vi "SelectMenu5.vi"(0 "XRef":T19, 1 "Tag":T14, 2 "Point":T17, 3 "Menu Type":T16, 4 "State In":T1) -> (14 "Reply":T13, 15 "Handled?":T15, 16 "Multi Object Popup Options":T12, 17 "Fatal Error Out":T11, 18 "State Out":T1)   [LabVIEW 2020, in "Parallel Diagram Block.xnode"]
uses:
  Parallel Diagram Block.xnode
  <vilib>/XNodeSupport/XNodeXNodeRef.ctl
  <vilib>/XNodeSupport/XNodeString.ctl
  <vilib>/XNodeSupport/XNodePoint.ctl
  <vilib>/XNodeSupport/XNodeInt.ctl
  <vilib>/XNodeSupport/XNodeMenuType.ctl
  State.ctl
  Parallel Block/Type Descriptor.ctl
  Parallel Block/Direction.ctl
  Parallel Block/Value Type.ctl
  Parallel Block/Terminal Mode.ctl
  Parallel Block/Terminal Type.ctl
  Parallel Block/Type Mode.ctl
  Parallel Block/Value Mode.ctl
  <vilib>/picture/picture.llb/imagedata.ctl
  Parallel Block/Manager Node.ctl
  <vilib>/XNodeSupport/XNodeStringArray.ctl
  <vilib>/XNodeSupport/XNodeBool.ctl
  <vilib>/XNodeSupport/XNodeMultiObjectPopupOptions.ctl
  <vilib>/XNodeSupport/XNodeErrorCluster.ctl
  Parallel Block/OpMenu Action.ctl
  Parallel Block/Parallel Block.lvlib
  <vilib>/XNodeSupport/NI_XNodeSupport.lvlib
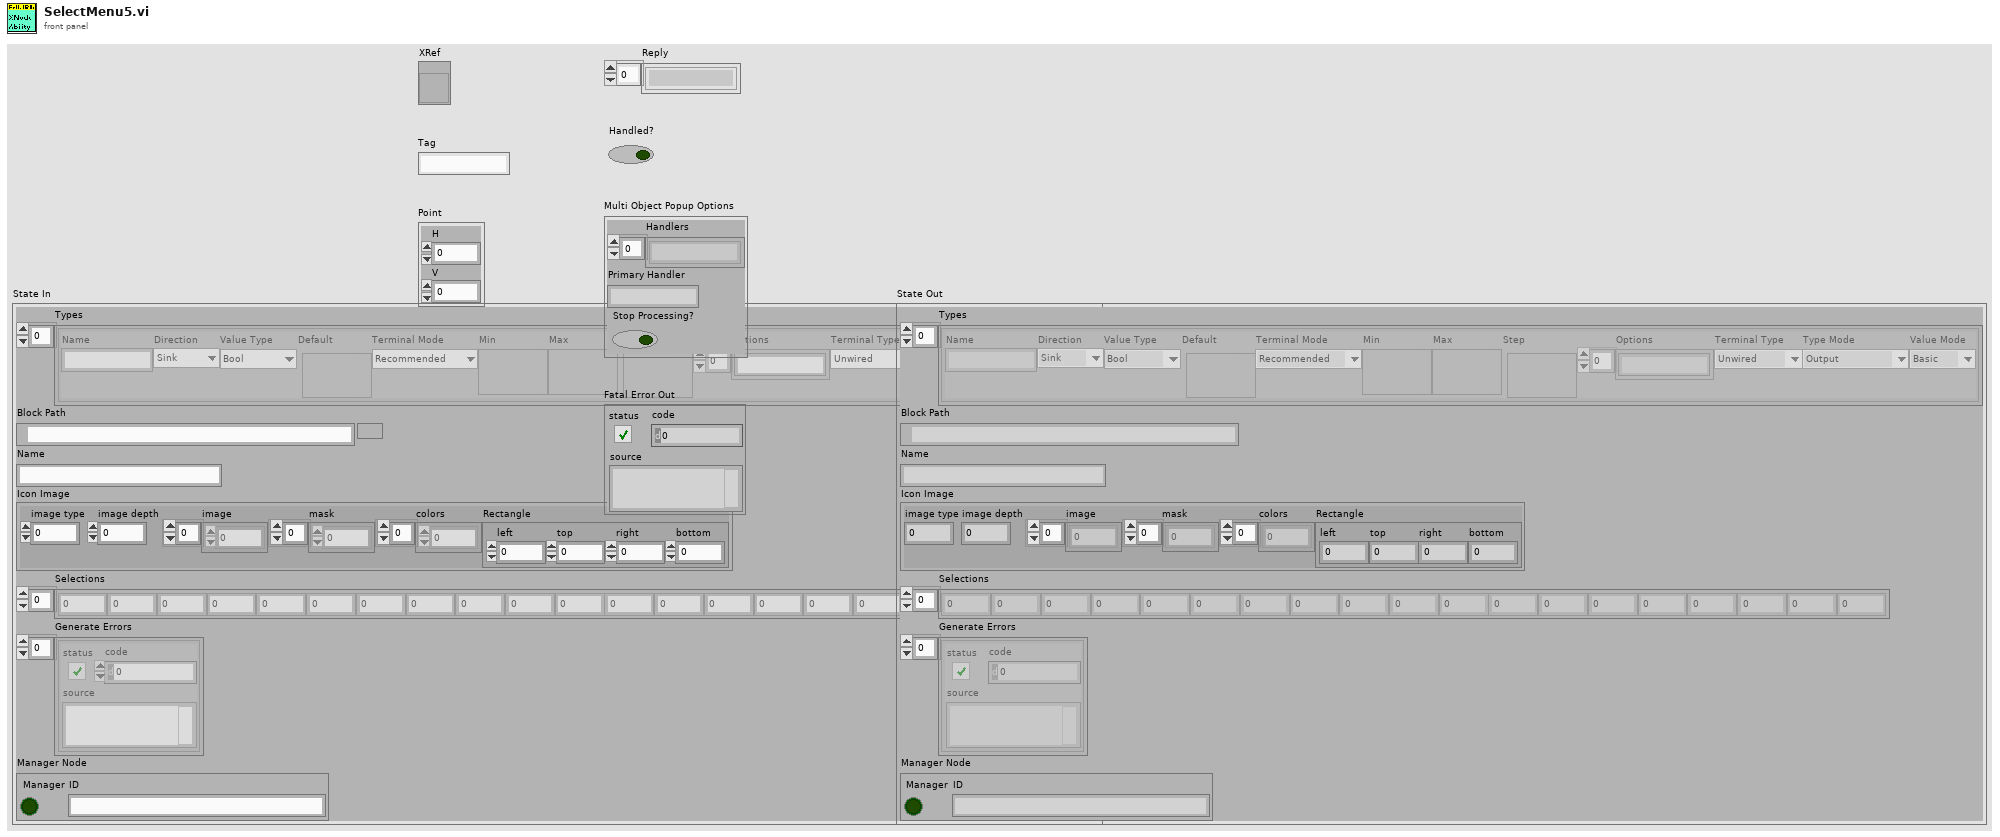
[diagram p1: front panel]
types:
  T1 = typedef "Parallel Diagram Block.xnode/State.ctl" = cluster{"Types":T2[], "Block Path":path, "Name":string, "Icon Image":T9, "Selections":i32[], "Generate Errors":errorcluster[], "Manager Node":T10}
  T2 = typedef "Parallel Block.lvlib/Type Descriptor.ctl" = cluster{"Name":string, "Direction":T3, "Value Type":T4, "Default":variant, "Terminal Mode":T5, "Min":variant, "Max":variant, "Step":variant, "Options":string[], "Terminal Type":T6, "Type Mode":T7, "Value Mode":T8}
  T3 = typedef "Parallel Block.lvlib/Direction.ctl" = enum16{"Sink", "Source"}
  T4 = typedef "Parallel Block.lvlib/Value Type.ctl" = enum16{"Unknown", "Bool", "U8", "U16", "U32", "U64", "I8", "I16", "I32", "I64", "SGL", "DBL", "CSG", "CDB", "CDBWfm", "String", "DBLWfm"}
  T5 = typedef "Parallel Block.lvlib/Terminal Mode.ctl" = enum16{"Recommended", "Required", "None"}
  T6 = typedef "Parallel Block.lvlib/Terminal Type.ctl" = enum16{"Unwired", "BadType", "Connection", "Value", "Control Ref", "BadRefType"}
  T7 = typedef "Parallel Block.lvlib/Type Mode.ctl" = enum16{"Output", "Single - Strict", "Single - Coerced", "Stream"}
  T8 = typedef "Parallel Block.lvlib/Value Mode.ctl" = enum16{"Basic", "Range", "Select"}
  T9 = typedef "imagedata.ctl" = cluster{"image type":i32, "image depth":i32, "image":u8[], "mask":u8[], "colors":u32[], "Rectangle":cluster{"left":i16, "top":i16, "right":i16, "bottom":i16}}
  T10 = typedef "Parallel Block.lvlib/Manager Node.ctl" = cluster{"Manager":bool, "ID":string}
  T11 = typedef "NI_XNodeSupport.lvlib/XNodeErrorCluster.ctl" = errorcluster
  T12 = typedef "NI_XNodeSupport.lvlib/XNodeMultiObjectPopupOptions.ctl" = cluster{"Handlers":T13, "Primary Handler":T14, "Stop Processing?":T15}
  T13 = typedef "NI_XNodeSupport.lvlib/XNodeStringArray.ctl" = T14[]
  T14 = typedef "NI_XNodeSupport.lvlib/XNodeString.ctl" = string
  T15 = typedef "NI_XNodeSupport.lvlib/XNodeBool.ctl" = bool
  T16 = typedef "NI_XNodeSupport.lvlib/XNodeMenuType.ctl" = enum32{"Single Object Operate", "Single Object Popup", "Multi Object Popup Master", "Multi Object Popup Other"}
  T17 = typedef "NI_XNodeSupport.lvlib/XNodePoint.ctl" = cluster{"H":T18, "V":T18}
  T18 = typedef "NI_XNodeSupport.lvlib/XNodeInt.ctl" = i32
  T19 = typedef "NI_XNodeSupport.lvlib/XNodeXNodeRef.ctl" = refnum<vi>
  T20 = typedef "Parallel Block.lvlib/OpMenu Action.ctl" = enum16{"Selector"}
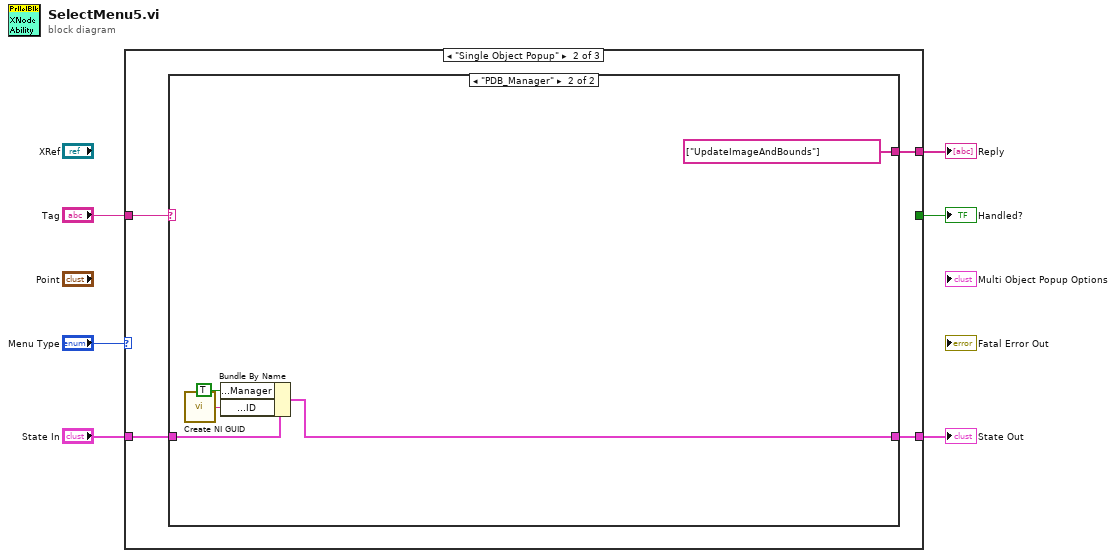
[diagram p0: block diagram]
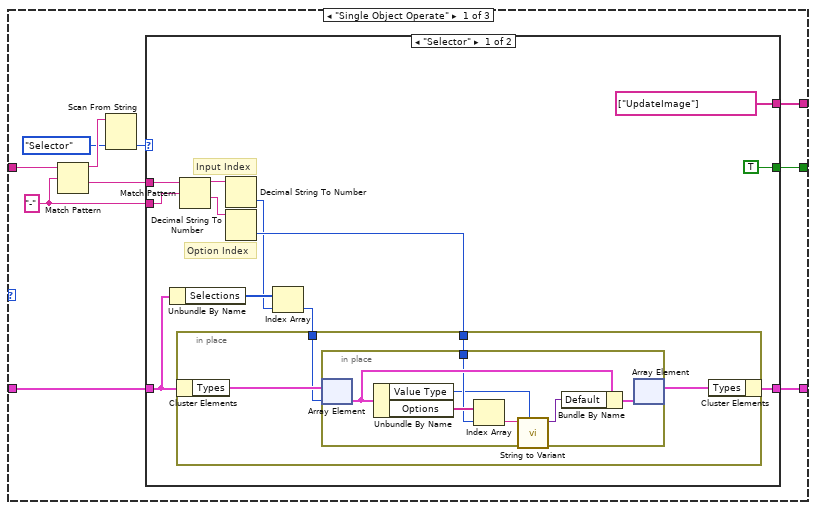
[diagram p2: hidden frame]
diagram:
  n1 = case shown="\"Single Object Popup\"" "Menu Type" {
    tunnel: "State In" -> [w10 w43 w51]
    tunnel: [w9 w42 w51] -> w5
    tunnel: "Tag" -> [w16 w44 _]
    tunnel: [w8 w41 _] -> w2
    tunnel: [w7 _ _] -> w1
    frame "Single Object Operate" {
      w11 = "-" ("regular expression")
      n2 = Match Pattern(string=w16, regular expression=w11) -> (before substring=w15:T14, after substring=w12:T14)  [unwired: 1 in, 2 out]
      n3 = Scan From String(input string=w15, default 1=OpMenu_Action."Selector" ("OpMenu Action")) -> (output 1=w13:T20)  [unwired: 3 in, 3 out]
      n4 = case shown="\"Selector\"" w13 {
        tunnel: w12 -> [w26 _]
        tunnel: w11 -> [w25 _]
        tunnel: w10 -> [w20 w40]
        tunnel: [w24 w40] -> w9
        tunnel: [string[] ["UpdateImage"] _] -> w8
        tunnel: [TRUE _] -> w7
        frame "Selector" {
          # "Option Index"
          # "Input Index"
          n5 = Unbundle By Name(w20) -> ("Selections"=w19:i32[])
          n6 = Match Pattern(string=w26, regular expression=w25) -> (before substring=w28:T14, after substring=w27:T14)  [unwired: 1 in, 2 out]
          n7 = Decimal String To Number(string=w28) -> (number=w18:i32)  [unwired: 2 in, 1 out]
          n8 = Decimal String To Number(string=w27) -> (number=w23:i32)  [unwired: 2 in, 1 out]
          n9 = Index Array(array=w19, index=w18) -> (element=w17:i32)
          n10 = in-place {
            in-place-border: w23 -> [w30]
            in-place-border: w17 -> [w29]
            n11 = in-place-cluster #1(w20) -> ("Types"=w32:T2[])
            n12 = in-place {
              in-place-border: w30 -> [w37]
              n13 = in-place-array #2(w32, w29) -> (w39:T2)
              n14 = Unbundle By Name(w39) -> ("Value Type"=w35:T4, "Options"=w38:string[])
              n15 = Index Array(array=w38, index=w37) -> (element=w36:string)
              n16 = call "String to Variant.vi"("Value Type"=w35, "String"=w36) -> ("Variant"=w34:variant)  [unwired: 7 in, 2 out]
              n17 = Bundle By Name(cluster=w39, "Default"=w34) -> (w33:T2)
              n18 = in-place-array #2(w33) -> (w31:T2[])  [unwired: 1 out]
            }
            n19 = in-place-cluster #1("Types"=w31) -> (w24:T1)
          }
        }
        frame Default {
        }
      }
    }
    frame "Single Object Popup" {
      n20 = case shown="\"PDB_Manager\"" w44 {
        tunnel: w43 -> [w45 w50]
        tunnel: [w45 w47] -> w42
        tunnel: [_ string[] ["UpdateImageAndBounds"]] -> w41
        frame Default {
        }
        frame "PDB_Manager" {
          n21 = call <vilib>:"Create NI GUID.vi"() -> ("NI GUID"=w48:string)
          n22 = Bundle By Name(cluster=w50, "Manager Node.Manager"=TRUE, "Manager Node.ID"=w48) -> (w47:T1)
        }
      }
    }
    frame Default {
    }
  }
  "Reply" <- w2
  "Handled?" <- w1
  "State Out" <- w5
